vi "Turret Structure.vi"(0 "AIDeviceRef":T1, 1 "Raw Turret":dbl, 2 "Left":dbl=4.5, 3 "Right":dbl=0.85, 5 "Turret Case":i32, 7 "Home Speed":dbl=1.0, 9 "Home postion":dbl, 11 "error in (no error)":errorcluster, 12 "Auton Right":dbl) -> (6 "Turret Output":dbl, 15 "Turret Case Output":dbl)   [LabVIEW 2011]
uses:
  <vilib>/Rock Robotics/WPI/AnalogChannel/WPI_AnalogChannelDevRef.ctl
  <vilib>/Rock Robotics/SystemInterfaces/Typedef/FPGA_TypedefAnalogModule.ctl
  <vilib>/Rock Robotics/SystemInterfaces/AI/FPGA_AIChannel.ctl
  <vilib>/addons/control/pid/pid.llb/PID (DBL).vi
  <vilib>/addons/control/pid/NI_PID_pid.lvlib
panel:
  in  "-1/1 per degree":dbl=0.05
  in  "Volts per degree":dbl=0.0166666666666667
  in  "PID Gains":T4={"proportional gain (Kc)"=1.0, "integral time (Ti, min)"=0.01, "derivative time (Td, min)"=0.0} {"derivative time (Td, min)" format="%.3f"; "integral time (Ti, min)" format="%.3f"; "proportional gain (Kc)" format="%.3f"}
  out "Waveform Chart":dynamicdata(graph)
  in  "PID Enable":bool
  # "Bring from Right to Left"
  # "Right Joystick moves Left"
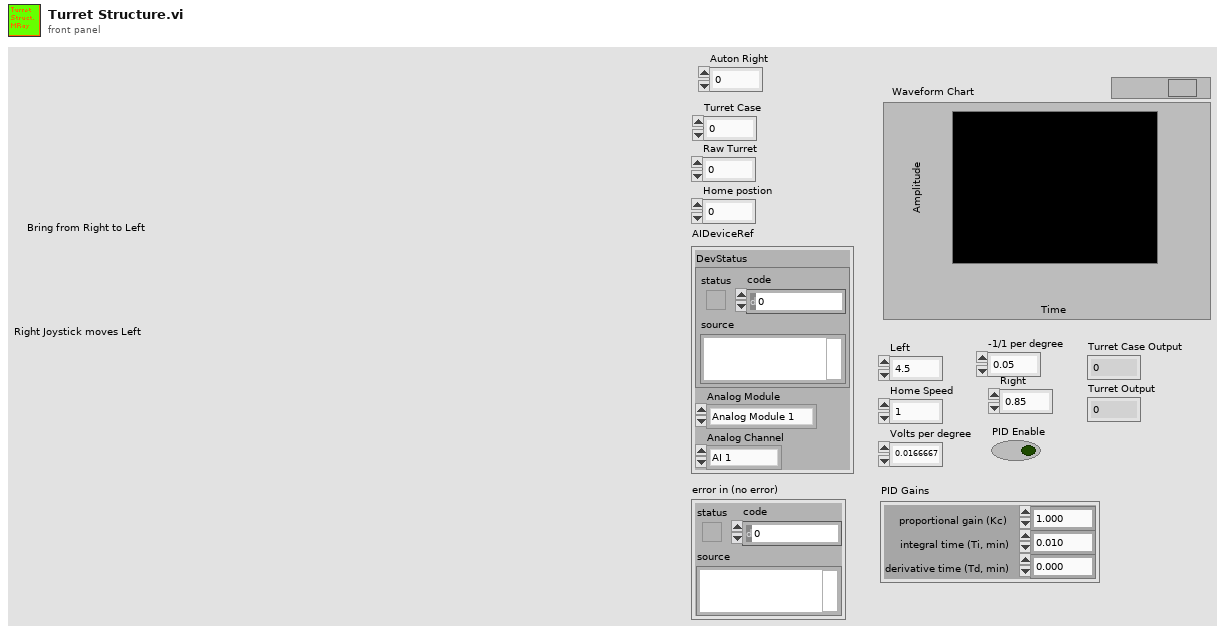
[diagram p1: front panel]
types:
  T1 = typedef "WPI_AnalogChannelDevRef.ctl" = cluster{"DevStatus":errorcluster, "Analog Module":T2, "Analog Channel":T3}
  T2 = typedef "FPGA_TypedefAnalogModule.ctl" = enum16{"Analog Module 1", "Analog Module 2"}
  T3 = typedef "FPGA_AIChannel.ctl" = enum8{"AI 1", "AI 2", "AI 3", "AI 4", "AI 5", "AI 6", "AI 7", "AI 8", "Invalid"}
  T4 = cluster{"proportional gain (Kc)":dbl, "integral time (Ti, min)":dbl, "derivative time (Td, min)":dbl}
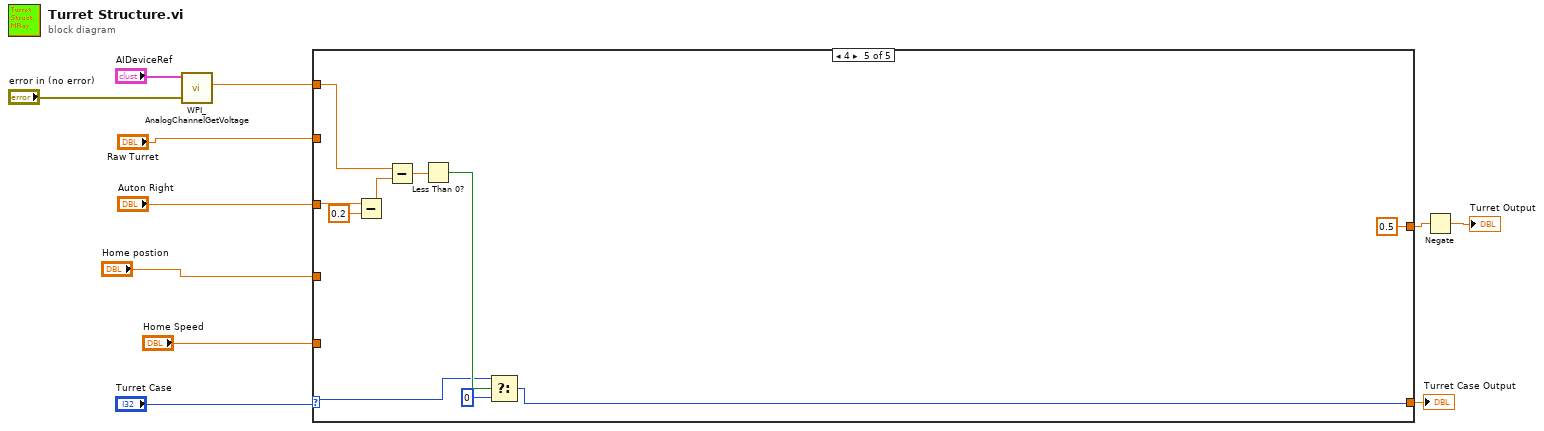
[diagram p0: block diagram]
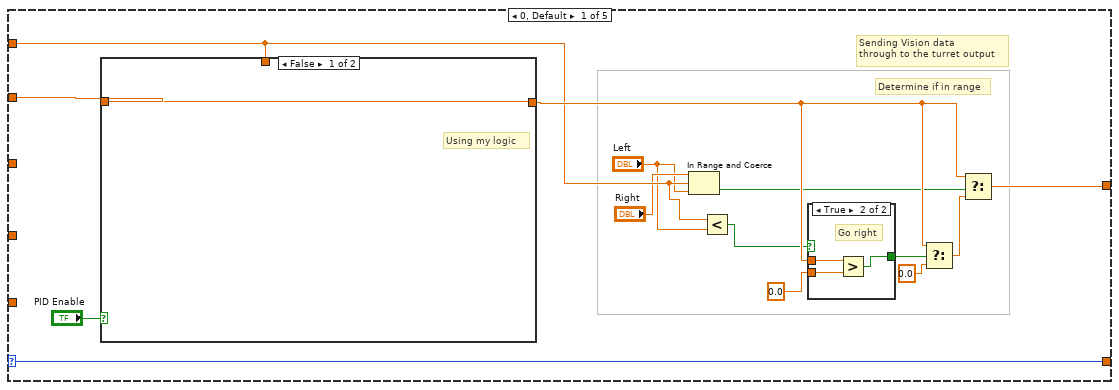
[diagram p2: hidden frame]
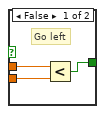
[diagram p3: hidden frame]
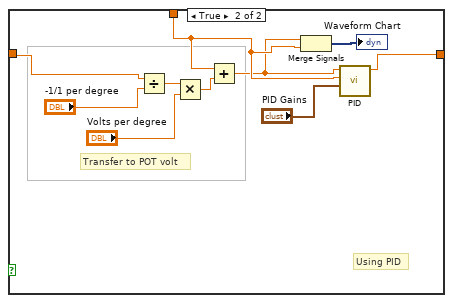
[diagram p4: hidden frame]
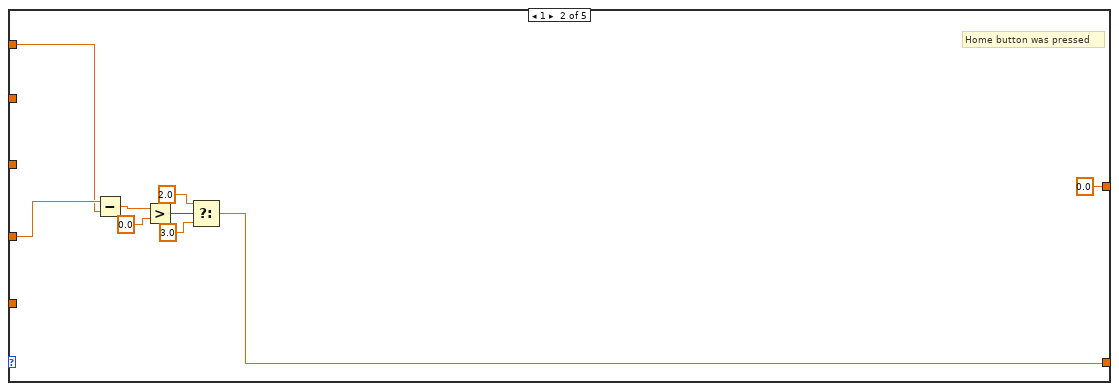
[diagram p5: hidden frame]
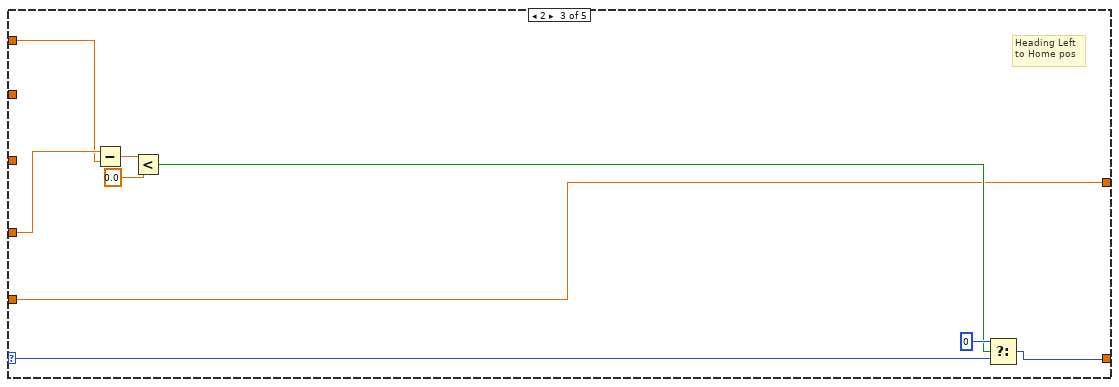
[diagram p6: hidden frame]
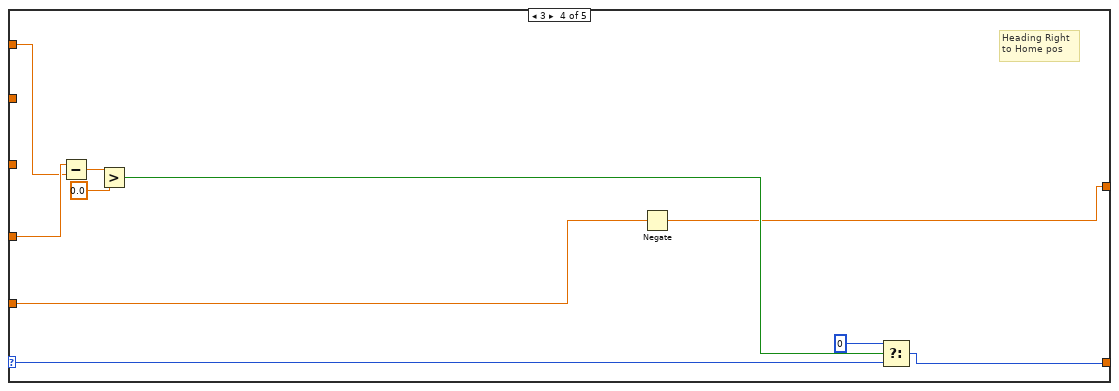
[diagram p7: hidden frame]
diagram:
  n1 = call <vilib>:"WPI_AnalogChannelGetVoltage.vi"("error in (no error)"="error in (no error)", "AIDeviceRef"="AIDeviceRef") -> ("Voltage"=w11:dbl)  [unwired: 7 in, 2 out]
  n2 = case shown="4" "Turret Case" {
    selector: "Turret Case" -> [w17 _ w56 w66 w77]
    tunnel: w11 -> [w16 w47 w52 w61 w80]
    tunnel: "Raw Turret" -> [w24 _ _ _ _]
    tunnel: [w18 0.0 ("Home Speed 2") w53 w62 0.5 ("Home Speed")] -> w3
    tunnel: "Home postion" -> [_ w48 w58 w68 _]
    tunnel: [w17 w46 w55 w65 w75] -> w4
    tunnel: "Home Speed" -> [_ _ w53 w63 _]
    tunnel: "Auton Right" -> [_ _ _ _ w74]
    frame 0, Default {
      # "Determine if in range"
      # "Sending Vision data\nthrough to the turret output"
      n3 = case shown="False" "PID Enable" {
        tunnel: w24 -> [w32 w41]
        tunnel: [w32 w36] -> w20
        tunnel: w16 -> [_ w34]
        frame False {
          # "Using my logic"
        }
        frame True {
          # "Transfer to POT volt"
          # "Using PID"
          n4 = Divide(x=w41, y="-1/1 per degree") -> (x/y=w40:dbl)
          n5 = Multiply(x=w40, y="Volts per degree") -> (x*y=w38:dbl)
          n6 = Add(x=w34, y=w38) -> (x+y=w33:dbl)
          n7 = Merge Signals(w33, w34) -> (→"Waveform Chart":dynamicdata)
          n8 = call-poly <vilib>:"PID.vi"("PID gains"="PID Gains", "process variable"=w34, "setpoint"=w33) -> ("output"=w36:dbl)  [unwired: 7 in, 1 out]
        }
      }
      n9 = In Range and Coerce(upper limit="Right", x=w16, lower limit="Left") -> (In Range?=w15:bool)  [unwired: 1 out]
      n10 = Less?(x=w16, y="Left") -> (x < y?=w12:bool)
      n11 = case shown="True" w12 {
        tunnel: 0.0 -> [w27 w31]
        tunnel: [w26 w30] -> w21
        tunnel: w20 -> [w28 w29]
        frame False {
          # "Go left"
          n12 = Less?(x=w28, y=w27) -> (x < y?=w26:bool)
        }
        frame True {
          # "Go right"
          n13 = Greater?(x=w29, y=w31) -> (0:w30:bool)
        }
      }
      n14 = Select(t=w20, s=w21, f=0.0) -> (s? t:f=w19:dbl)
      n15 = Select(t=w20, s=w15, f=w19) -> (s? t:f=w18:dbl)
    }
    frame 1 {
      # "Home button was pressed"
      n16 = Subtract(x=w48, y=w47) -> (x-y=w49:dbl)
      n17 = Greater?(x=w49, y=0.0) -> (0:w51:bool)
      n18 = Select(t=2.0, s=w51, f=3.0) -> (s? t:f=w46:dbl)
    }
    frame 2 {
      # "Heading Left\nto Home pos"
      n19 = Subtract(x=w58, y=w52) -> (x-y=w59:dbl)
      n20 = Less?(x=w59, y=0.0) -> (x < y?=w54:bool)
      n21 = Select(t=0, s=w54, f=w56) -> (s? t:f=w55:i32)
    }
    frame 3 {
      # "Heading Right\nto Home pos"
      n22 = Subtract(x=w68, y=w61) -> (x-y=w69:dbl)
      n23 = Greater?(x=w69, y=0.0) -> (0:w64:bool)
      n24 = Negate(x=w63) -> (-x=w62:dbl)
      n25 = Select(t=0, s=w64, f=w66) -> (s? t:f=w65:i32)
    }
    frame 4 {
      n26 = Subtract(x=w74, y=0.2) -> (x-y=w72:dbl)
      n27 = Subtract(x=w80, y=w72) -> (x-y=w79:dbl)
      n28 = Less Than 0?(x=w79) -> (x < 0?=w78:bool)
      n29 = Select(t=w77, s=w78, f=0) -> (s? t:f=w75:i32)
    }
  }
  "Turret Case Output" <- w4
  n30 = Negate(x=w3) -> (-x=→"Turret Output":dbl)
